vi "FSRS Experiments Form.vi"() -> ()   [LabVIEW 2020]
uses:
  source/Field/Field.lvclass
  source/ODBC/ADODB.lvclass
  C:/Users/User/Desktop/Raman Program/Database OOP/source/Database/Database.lvclass
  source/Field/FK Ring Field Info.ctl
  source/FK Ring/FK Ring Info.ctl
  source/Field/Text Field Info.ctl
  source/Field/Field.lvclass/Field.ctl
  source/Field/Constructor by Info Cluster FK Ring.vi
  source/Field/Constructor by Info Cluster Text.vi
  source/Database/Database.lvclass
  C:/Users/User/Desktop/Raman Program/Database OOP/source/ODBC/ADODB.lvclass
panel:
  out "Label.Text":string
  in  "stop":bool
  in  "OK Button":bool
  in  "Working Range":u16(ring) items=["None"=1]
  in  "Description":string
  in  "Sample":u16(ring) items=["None"=1, "P"=2, "BSP"=3, "R"=4, "OC"=5, "undoped"=6, "A"=7, "S"=8]
  in  "Data Set":u16(ring) items=["Chopper Phase"=1, "Solvent GS Raman"=2, "Raman Chirp Test"=3, "STO GS Raman"=4, "Program Test"=5, "Front vs Back Refl"=6, "OC ES Raman"=7, "CC ES Raman"=8, "Interfacial Water Test"=9]
  in  "User":u16(ring) items=["None"=1, "Michael"=2, "Suryansh"=3, "Ilya"=4, "Hanna"=5, "Tanja"=6]
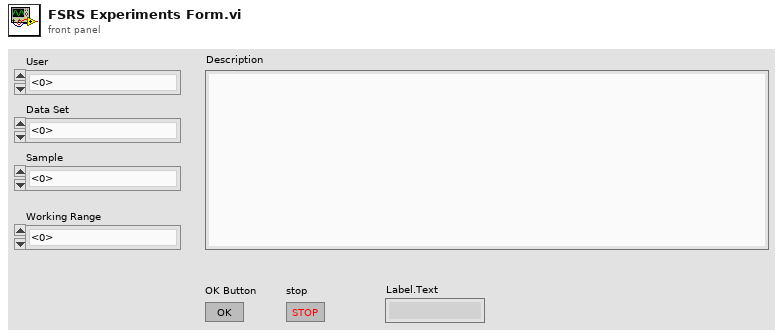
[diagram p1: front panel]
types:
  T1 = typedef "FK Ring Field Info.ctl" = cluster{"Ctl Refnum":refnum<vi>, "FK Table":string, "FK Column":string, "FK Ring Info":T2}
  T2 = typedef "FK Ring Info.ctl" = cluster{"PK Table":string, "PK Column":string, "PK Display Column":string}
  T3 = typedef "Text Field Info.ctl" = cluster{"Ctl Refnum":refnum<vi>, "Table":string, "Column":string}
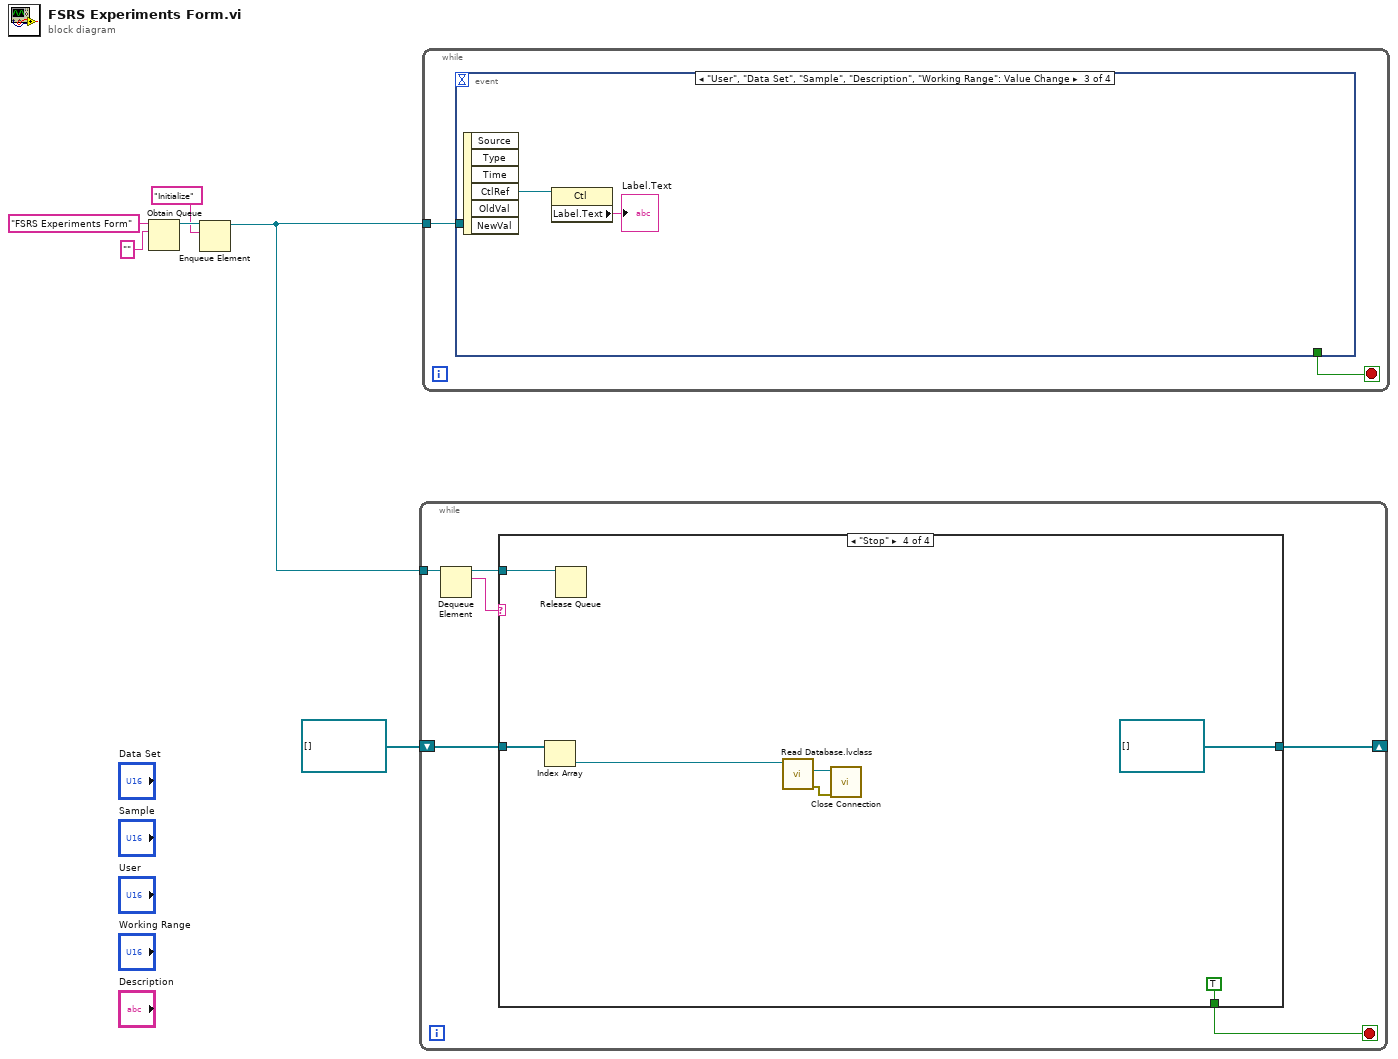
[diagram p0: block diagram]
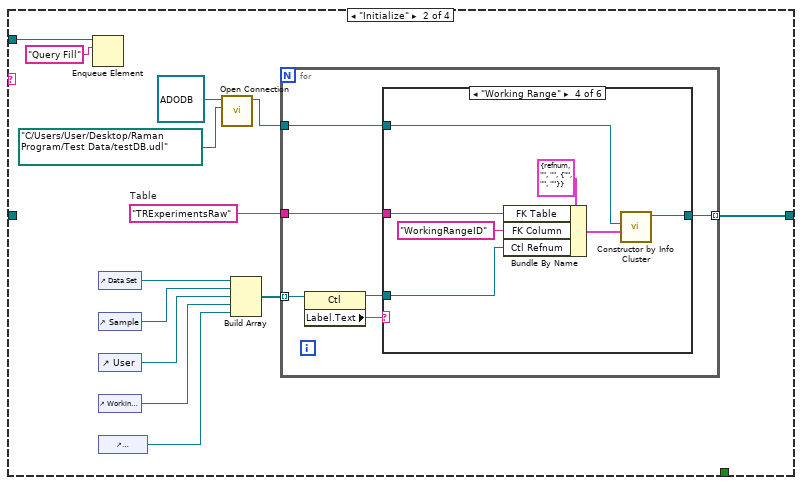
[diagram p3: hidden frame]
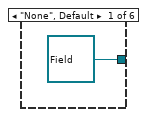
[diagram p4: hidden frame]
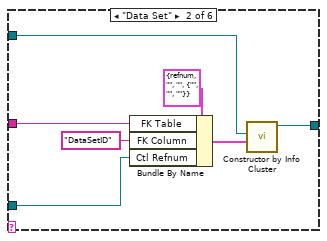
[diagram p5: hidden frame]
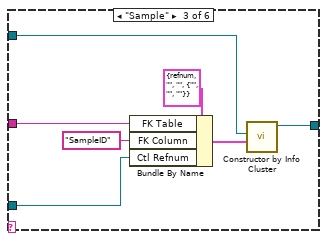
[diagram p6: hidden frame]
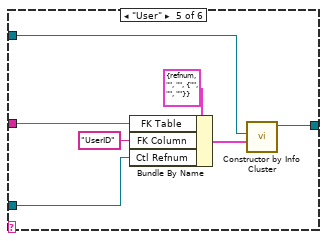
[diagram p7: hidden frame]
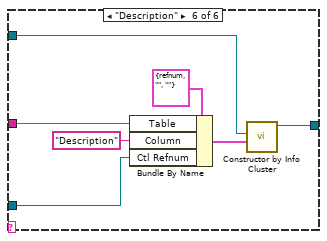
[diagram p8: hidden frame]
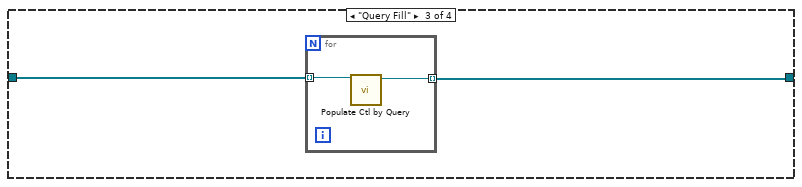
[diagram p9: hidden frame]
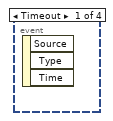
[diagram p10: hidden frame]
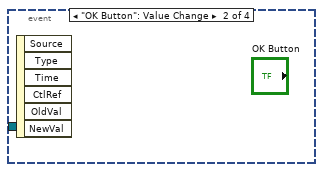
[diagram p11: hidden frame]
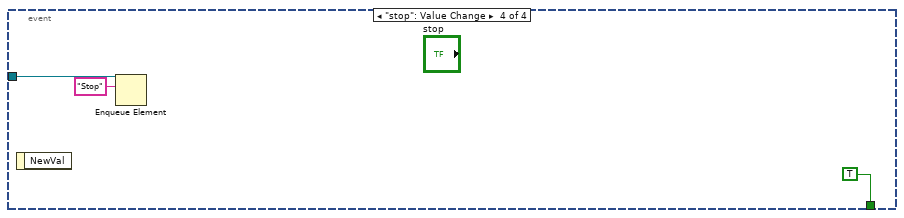
[diagram p12: hidden frame]
diagram:
  n1 = Obtain Queue(name (unnamed)="FSRS Experiments Form", element data type="") -> (queue out=w5:refnum<queue>)  [unwired: 3 in, 2 out]
  n2 = Enqueue Element(queue=w5, element="Initialize") -> (queue out=w2:refnum<queue>)  [unwired: 2 in, 2 out]
  n3 = while {
    shift-right: [w12] -> _
    shift-left: refnum<class "Field.lvclass">[] [] -> [w11]
    tunnel: w2 -> [w9]
    stop <- w8 stop-if-true
    n4 = Dequeue Element(queue=w9) -> (queue out=w7:refnum<queue>, element=w10:string)  [unwired: 2 in, 2 out]
    n5 = case shown="\"Stop\"" w10 {
      tunnel: [w13 w20 w69 refnum<class "Field.lvclass">[] []] -> w12
      tunnel: w11 -> [w13 _ w70 w76]
      tunnel: [_ _ _ TRUE] -> w8
      tunnel: w7 -> [_ w15 _ w74]
      frame "None", Default {
      }
      frame "Initialize" {
        w19 = "TRExperimentsRaw"  # Table
        n6 = Enqueue Element(queue=w15, element="Query Fill") -> ()  [unwired: 2 in, 3 out]
        n7 = control-ref of="Data Set"() -> (w26:refnum<vi>)
        n8 = control-ref of="Sample"() -> (w25:refnum<vi>)
        n9 = control-ref of="User"() -> (w23:refnum<vi>)
        n10 = control-ref of="Working Range"() -> (w22:refnum<vi>)
        n11 = control-ref of="Description"() -> (w21:refnum<vi>)
        n12 = call-dynamic "Open Connection.vi"("Connection Info (Member Data/Prompt)"=path "C:/Users/User/Desktop/Raman Program/Test Data/testDB.udl", "ODBC in"=refnum<class "ADODB.lvclass"> refnum) -> ("ODBC out"=w16:refnum<class "ADODB.lvclass">)  [unwired: 8 in, 1 out]
        n13 = Build Array(w26, w25, w23, w22, w21) -> (w24:refnum<vi>[])
        n14 = for {
          tunnel: w24 -> [w32] mode=indexing
          tunnel: w16 -> [w31]
          tunnel: w19 -> [w29]
          tunnel: [w27] -> w20 mode=indexing
          n15 = property class="Ctl"(reference=w32) -> (reference out=w30:refnum<vi>, "Label.Text"=w28:string)  [unwired: 1 in, 1 out]
          n16 = case shown="\"Working Range\"" w28 {
            tunnel: w31 -> [_ w40 w47 w54 w61 w68]
            tunnel: [refnum<class "Field.lvclass"> refnum ("Field out") w39 w46 w53 w60 w67] -> w27
            tunnel: w30 -> [_ w36 w43 w50 w57 w66]
            tunnel: w29 -> [_ w35 w42 w49 w56 w65]
            frame "None", Default {
            }
            frame "Data Set" {
              n17 = Bundle By Name(cluster=T1 {"Ctl Refnum"=refnum, "FK Table"="", "FK Column"="", "FK Ring Info"={"PK Table"="", "PK Column"="", "PK Display Column"=""}} ("FK Ring Field Info"), "FK Table"=w35, "FK Column"="DataSetID", "Ctl Refnum"=w36) -> (w37:T1)
              n18 = call-poly "Constructor by Info Cluster.vi"("FK Ring Field Info"=w37, "Database (use member data)"=w40) -> ("Field out"=w39:refnum<class "Field.lvclass">)  [unwired: 8 in, 1 out]
            }
            frame "Sample" {
              n19 = Bundle By Name(cluster=T1 {"Ctl Refnum"=refnum, "FK Table"="", "FK Column"="", "FK Ring Info"={"PK Table"="", "PK Column"="", "PK Display Column"=""}} ("FK Ring Field Info"), "FK Table"=w42, "FK Column"="SampleID", "Ctl Refnum"=w43) -> (w44:T1)
              n20 = call-poly "Constructor by Info Cluster.vi"("FK Ring Field Info"=w44, "Database (use member data)"=w47) -> ("Field out"=w46:refnum<class "Field.lvclass">)  [unwired: 8 in, 1 out]
            }
            frame "Working Range" {
              n21 = Bundle By Name(cluster=T1 {"Ctl Refnum"=refnum, "FK Table"="", "FK Column"="", "FK Ring Info"={"PK Table"="", "PK Column"="", "PK Display Column"=""}} ("FK Ring Field Info"), "FK Table"=w49, "FK Column"="WorkingRangeID", "Ctl Refnum"=w50) -> (w51:T1)
              n22 = call-poly "Constructor by Info Cluster.vi"("FK Ring Field Info"=w51, "Database (use member data)"=w54) -> ("Field out"=w53:refnum<class "Field.lvclass">)  [unwired: 8 in, 1 out]
            }
            frame "User" {
              n23 = Bundle By Name(cluster=T1 {"Ctl Refnum"=refnum, "FK Table"="", "FK Column"="", "FK Ring Info"={"PK Table"="", "PK Column"="", "PK Display Column"=""}} ("FK Ring Field Info"), "FK Table"=w56, "FK Column"="UserID", "Ctl Refnum"=w57) -> (w58:T1)
              n24 = call-poly "Constructor by Info Cluster.vi"("FK Ring Field Info"=w58, "Database (use member data)"=w61) -> ("Field out"=w60:refnum<class "Field.lvclass">)  [unwired: 8 in, 1 out]
            }
            frame "Description" {
              n25 = Bundle By Name(cluster=T3 {"Ctl Refnum"=refnum, "Table"="", "Column"=""} ("Text Field Info"), "Table"=w65, "Column"="Description" ("FK Column"), "Ctl Refnum"=w66) -> (w62:T3)
              n26 = call-poly "Constructor by Info Cluster.vi"("Text Field Info"=w62, "Database (use member data)"=w68) -> ("Field out"=w67:refnum<class "Field.lvclass">)  [unwired: 8 in, 1 out]
            }
          }
        }
      }
      frame "Query Fill" {
        n27 = for {
          tunnel: w70 -> [w72] mode=indexing
          tunnel: [w71] -> w69 mode=indexing
          n28 = call-dynamic "Populate Ctl by Query.vi"("Field in"=w72) -> ("Field out"=w71:refnum<class "Field.lvclass">)  [unwired: 9 in, 1 out]
        }
      }
      frame "Stop" {
        n29 = Index Array(array=w76) -> (element=w75:refnum<class "Field.lvclass">)  [unwired: 1 in]
        n30 = Release Queue(queue=w74) -> ()  [unwired: 2 in, 3 out]
        n31 = call "Read Database.lvclass.vi"("Field in"=w75) -> ("error out"=w79:errorcluster, "Database.lvclass"=w78:refnum<class "Database.lvclass">)  [unwired: 8 in, 1 out]
        n32 = call-dynamic "Close Connection.vi"("error in (no error)"=w79, "Database in"=w78) -> ()  [unwired: 8 in, 2 out]
      }
    }
  }
  n33 = while {
    tunnel: w2 -> [w81]
    stop <- w80 stop-if-true
    n34 = event shown="[2] \"User\", \"Data Set\", \"Sample\", \"Description\", \"Working Range\": Value Change" {
      selector: _ -> [_ _ _ _]
      dyn-events: _ -> [_ _ _ _]
      timeout: _ -> [_ _ _ _]
      tunnel: w81 -> [_ _ _ w86]
      tunnel: [_ _ _ TRUE] -> w80
      event Timeout {
        n35 = event-data() -> ()  [unwired: 1 in, 3 out]
      }
      event "OK Button": Value Change {
        n36 = event-data() -> ()  [unwired: 1 in, 6 out]
      }
      event "User", "Data Set", "Sample", "Description", "Working Range": Value Change {
        n37 = event-data() -> ("CtlRef"=w83:refnum<vi>)  [unwired: 1 in, 5 out]
        n38 = property class="Ctl"(reference=w83) -> ("Label.Text"=→"Label.Text":string)  [unwired: 1 in, 2 out]
      }
      event "stop": Value Change {
        n39 = event-data() -> ()  [unwired: 1 in, 1 out]
        n40 = Enqueue Element(queue=w86, element="Stop") -> ()  [unwired: 2 in, 3 out]
      }
    }
  }
